vi "Override Error.vi"(10 "Error":errorcluster, 11 "Override Error in":refnum<class "Override Error.lvclass">) -> (3 "Override Error out":refnum<class "Override Error.lvclass">)   [LabVIEW 2021, in "jettl Msg Override Error.lvlib" / "Override Error.lvclass"]
uses:
  Override Error.lvclass
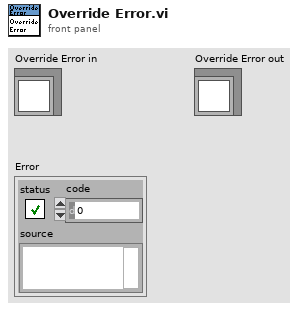
[diagram p1: front panel]
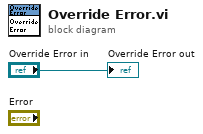
[diagram p0: block diagram]
diagram:
  "Override Error out" <- "Override Error in"
